vi "calc_addC_C345.vi"(9 "Add to C":dbl, 11 "Input U8":u8) -> (3 "Output U8":u8)   [LabVIEW 2018]
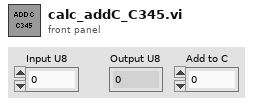
[diagram p1: front panel]
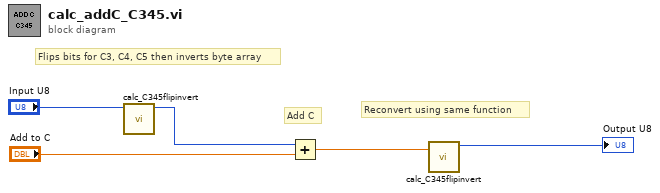
[diagram p0: block diagram]
diagram:
  # "Reconvert using same function"
  # "Add C"
  # "Flips bits for C3, C4, C5 then inverts byte array"
  n1 = call "calc_C345flipinvert.vi"("Input U8"="Input U8") -> ("Output U8"=w3:u8)  [unwired: 10 in]
  n2 = Add(x=w3, y="Add to C") -> (x+y=w2:dbl)
  n3 = call "calc_C345flipinvert.vi"("Input U8"=w2) -> ("Output U8"=→"Output U8":u8)  [unwired: 10 in]
